vi "Check Stopped.vi"(8 "error in (no error)":errorcluster, 11 "TCP Comm In":T1) -> (0 "error out":errorcluster, 2 "Stopped?":bool)   [LabVIEW 2020, in "TCP Comms.lvlib"]
uses:
  TCP Comms.lvlib
  State.ctl
  Ref Data.ctl
  TCP Comm.ctl
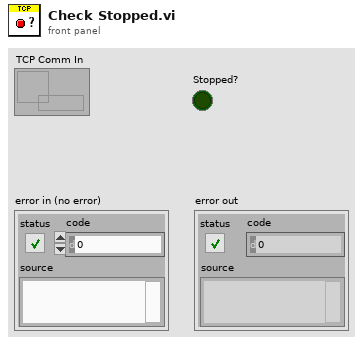
[diagram p1: front panel]
types:
  T1 = typedef "TCP Comms.lvlib/TCP Comm.ctl" = refnum<data-value>
  T2 = typedef "TCP Comms.lvlib/State.ctl" = enum16{"Idle", "Starting", "Connecting", "Connected", "Disconnecting", "Stopped"}
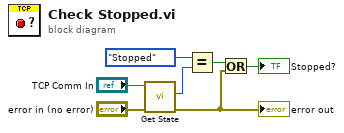
[diagram p0: block diagram]
diagram:
  n1 = call "Get State.vi"("error in (no error)"="error in (no error)", "TCP Comm In"="TCP Comm In") -> ("error out"=w2:errorcluster, "State"=w5:T2)  [unwired: 8 in]
  "error out" <- w2
  n2 = Equal?(x=State."Stopped", y=w5) -> (x = y?=w3:bool)
  n3 = Or(x=w3, y=w2) -> (x .or. y?=→"Stopped?":bool)
